vi "SAOMM-PositionGUI.vi"(0 "Hexapod VRN":refnum<visa-resource-name>="COM4", 1 "Active Refnum":refnum<vi>, 2 "PrAMS-ACK":refnum<vi>, 7 "output cluster":T1, 13 "MessageType":cluster{string[], u32[]}={["emtError", "emtAreYouThere", "emtAcknowledgment", "emtGetClientType", "emtClientType", "emtGetImageExposureTime", "emtSetImageExposureTime", "emtImageExposureTime", "emtGetOptimalExposureTime", "emtSetOptimalExposureTime", "emtOptimalExposureTime", "emtGetImageEMGain", "emtSetImageEMGain", "emtImageEMGain", "emtGetFPGACtrl", "emtSetFPGACtrl", "emtFPGACtrl", "emtGetImageWidth", "emtSetImageWidth", "emtImageWidth", "emtGetImageHeight", "emtSetImageHeight", "emtImageHeight", "emtGetImageBinning", "emtSetImageBinning", "emtImageBinning", "emtGetImageDisplayFrameRate", "emtSetImageDisplayFrameRate", "emtImageDisplayFrameRate", "emtGetROIWidth", "emtSetROIWidth", "emtROIWidth", "emtGetROIHeight", "emtSetROIHeight", "emtROIHeight", "emtGetROIXOffset", "emtSetROIXOffset", "emtROIXOffset", "emtGetROIYOffset", "emtSetROIYOffset", "emtROIYOffset", "emtStartAcquisition", "mtStopAcquisition", "emtAcquisitionStarted", "emtAcquisitionStopped", "emtGetFalconImage", "emtFalconImage"], [1, 2, 3, 4, 5, 1001, 1101, 1201, 1002, 1102, 1202, 1003, 1103, 1203, 1004, 1104, 1204, 1005, 1105, 1205, 1006, 1106, 1206, 1007, 1107, 1207, 1008, 1108, 1208, 1009, 1109, 1209, 1010, 1110, 1210, 1011, 1111, 1211, 1012, 1112, 1212, 1130, 1131, 1150, 1151, 1070, 1270]}) -> (8 "Error":bool)   [LabVIEW 2011]
uses:
  Polymorphics/Num2littleEndian(DBL).vi
panel:
  out "First Run":bool
  in  "Incrément":dbl
  in  "Incrément":dbl
  in  "V+":bool
  in  "V-":bool
  in  "U+":bool
  in  "Cancel 8":bool
  in  "Cancel 7":bool
  in  "Cancel 6":bool
  in  "Cancel 5":bool
  in  "Cancel 4":bool
  in  "Cancel 3":bool
  in  "X-":bool
  in  "keep-active":bool caption="Laisser ouvert ?"
  in  "Signature":u32=1886544237
  in  "Cancel":bool
  in  "Send":bool
  in  "X":dbl caption="Pos" format="%.4f"
  in  "Y":dbl caption="Pos" format="%.4f"
  in  "Z":dbl caption="Pos" format="%.4f"
  in  "U":dbl caption="Pos" format="%.4f"
  in  "V":dbl caption="Pos" format="%.4f"
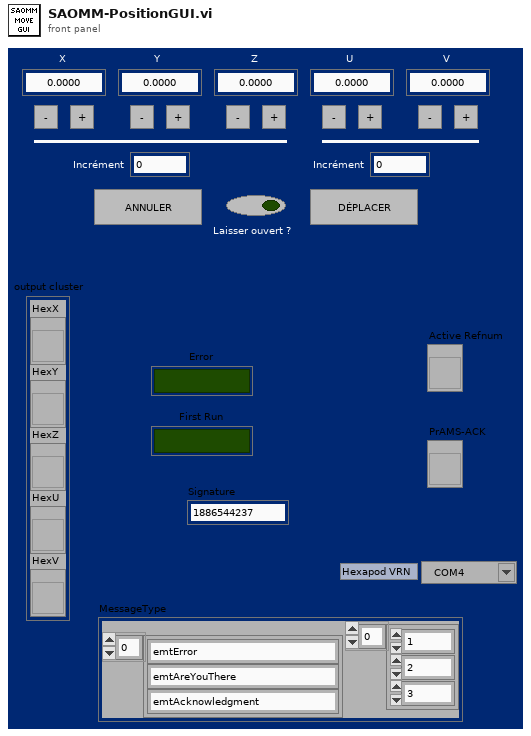
[diagram p1: front panel]
types:
  T1 = cluster{"HexX":refnum<vi>, "HexY":refnum<vi>, "HexZ":refnum<vi>, "HexU":refnum<vi>, "HexV":refnum<vi>}
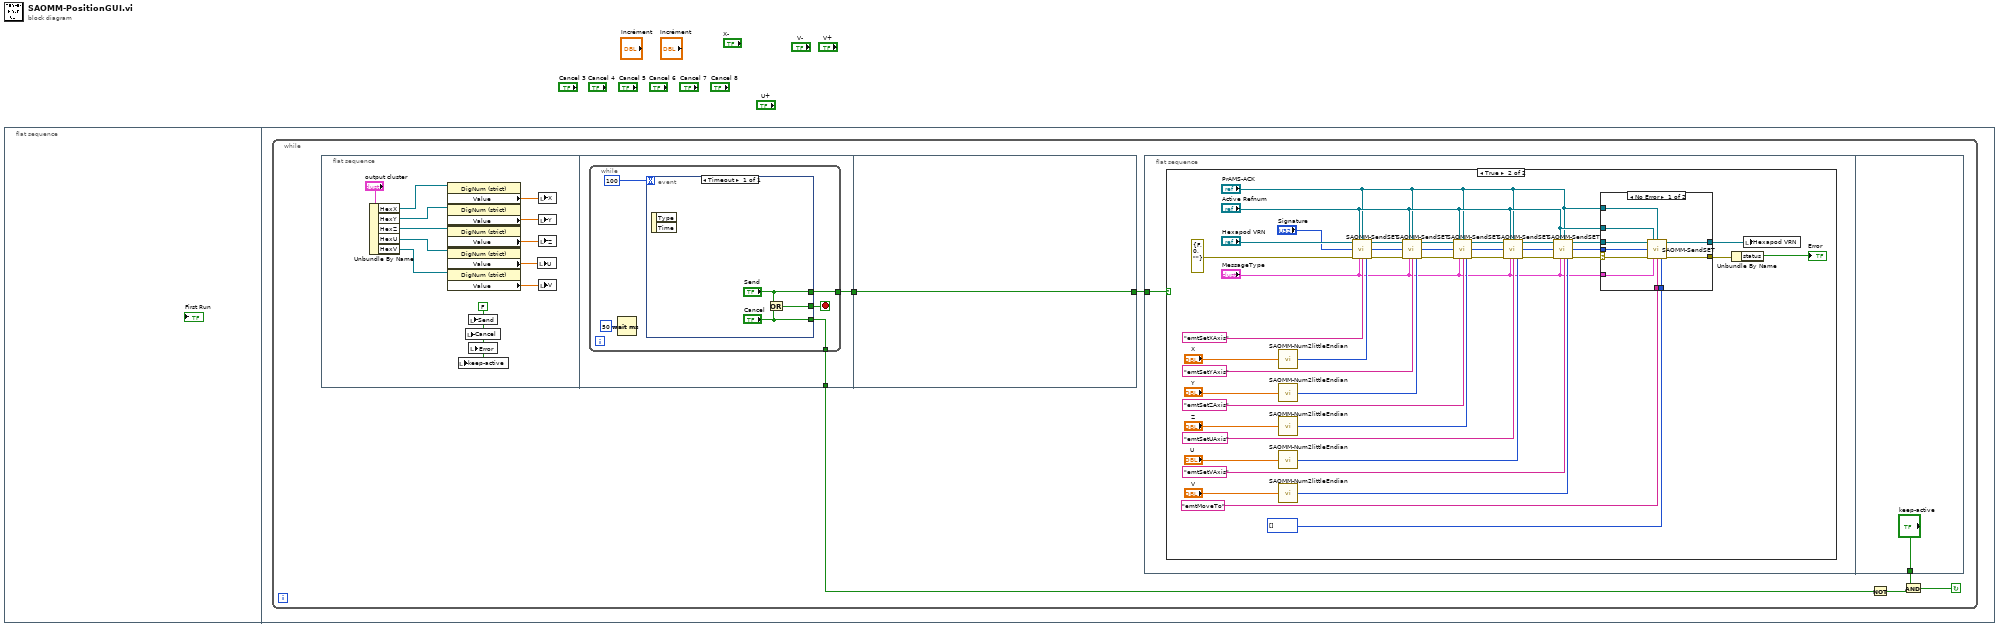
[diagram p0: block diagram]
diagram:
  n1 = flat-sequence {
    frame #0 {
    }
    frame #1 {
      n2 = while {
        stop <- w4 continue-if-true
        n3 = flat-sequence {
          tunnel: [w69] -> w2
          tunnel: [w70] -> w1
          tunnel: [w79] -> w6
          tunnel: w1 -> [w79]
          frame #0 {
            w57 = FALSE
            n4 = Unbundle By Name("output cluster") -> ("HexX"=w67:refnum<vi>, "HexY"=w66:refnum<vi>, "HexZ"=w65:refnum<vi>, "HexU"=w64:refnum<vi>, "HexV"=w63:refnum<vi>)
            n5 = property class="DigNum (strict)"(reference=w67) -> ("Value"=w58:dbl)  [unwired: 1 in, 2 out]
            n6 = property class="DigNum (strict)"(reference=w66) -> ("Value"=w59:dbl)  [unwired: 1 in, 2 out]
            n7 = property class="DigNum (strict)"(reference=w65) -> ("Value"=w60:dbl)  [unwired: 1 in, 2 out]
            n8 = property class="DigNum (strict)"(reference=w64) -> ("Value"=w61:dbl)  [unwired: 1 in, 2 out]
            n9 = property class="DigNum (strict)"(reference=w63) -> ("Value"=w62:dbl)  [unwired: 1 in, 2 out]
            n10 = local write "keep-active"(w57) -> ()
            n11 = local write "Cancel"(w57) -> ()
            n12 = local write "Send"(w57) -> ()
            n13 = local write "Error"(w57) -> ()
            n14 = local write "U"(w61) -> ()
            n15 = local write "X"(w58) -> ()
            n16 = local write "Y"(w59) -> ()
            n17 = local write "Z"(w60) -> ()
            n18 = local write "V"(w62) -> ()
          }
          frame #1 {
            n19 = while {
              tunnel: [w72] -> w70
              tunnel: [w71] -> w69
              stop <- w73 stop-if-true
              n20 = Wait (ms)(milliseconds to wait=u32 50) -> ()  [unwired: 1 out]
              n21 = event shown="[0] Timeout" {
                selector: _ -> [_]
                dyn-events: _ -> [_]
                timeout: 100 -> [_]
                tunnel: [w78] -> w73
                tunnel: ["Send"] -> w72
                tunnel: ["Cancel"] -> w71
                event Timeout {
                  n22 = event-data() -> ()  [unwired: 1 in, 2 out]
                  n23 = Or(x="Send", y="Cancel") -> (x .or. y?=w78:bool)
                }
              }
            }
          }
          frame #2 {
          }
        }
        n24 = flat-sequence {
          tunnel: w6 -> [w7]
          tunnel: ["keep-active"] -> w5
          frame #0 {
            n25 = case shown="True" w7 {
              frame False {
              }
              frame True {
                n26 = call-poly "SAOMM-Num2littleEndian.vi"("Number"="X") -> ("LiitleEndianedData"=w30:u8[])  [unwired: 14 in]
                n27 = call-poly "SAOMM-Num2littleEndian.vi"("Number"="Y") -> ("LiitleEndianedData"=w31:u8[])  [unwired: 14 in]
                n28 = call-poly "SAOMM-Num2littleEndian.vi"("Number"="Z") -> ("LiitleEndianedData"=w32:u8[])  [unwired: 14 in]
                n29 = call-poly "SAOMM-Num2littleEndian.vi"("Number"="U") -> ("LiitleEndianedData"=w35:u8[])  [unwired: 14 in]
                n30 = call-poly "SAOMM-Num2littleEndian.vi"("Number"="V") -> ("LiitleEndianedData"=w36:u8[])  [unwired: 14 in]
                n31 = call "SAOMM-SendSET.vi"("PRAMMS-COMM IN"="Hexapod VRN", "Active Refnum"="Active Refnum", "PrAMS-ACK"="PrAMS-ACK", "Signature"="Signature", "Error IN"=errorcluster {"status"=FALSE, "code"=0, "source"=""}, "MessageType"="MessageType", "Active SET"="emtSetXAxis", "Value (little endianed byte array)"=w30) -> ("PRAMMS-COMM OUT"=w21:refnum<visa-resource-name>, "Error OUT"=w27:errorcluster)  [unwired: 4 in, 2 out]
                n32 = call "SAOMM-SendSET.vi"("PRAMMS-COMM IN"=w21, "Active Refnum"="Active Refnum", "PrAMS-ACK"="PrAMS-ACK", "Signature"="Signature", "Error IN"=w27, "MessageType"="MessageType", "Active SET"="emtSetYAxis", "Value (little endianed byte array)"=w31) -> ("PRAMMS-COMM OUT"=w22:refnum<visa-resource-name>, "Error OUT"=w26:errorcluster)  [unwired: 4 in, 2 out]
                n33 = call "SAOMM-SendSET.vi"("PRAMMS-COMM IN"=w22, "Active Refnum"="Active Refnum", "PrAMS-ACK"="PrAMS-ACK", "Signature"="Signature", "Error IN"=w26, "MessageType"="MessageType", "Active SET"="emtSetZAxis", "Value (little endianed byte array)"=w32) -> ("PRAMMS-COMM OUT"=w42:refnum<visa-resource-name>, "Error OUT"=w25:errorcluster)  [unwired: 4 in, 2 out]
                n34 = call "SAOMM-SendSET.vi"("PRAMMS-COMM IN"=w42, "Active Refnum"="Active Refnum", "PrAMS-ACK"="PrAMS-ACK", "Signature"="Signature", "Error IN"=w25, "MessageType"="MessageType", "Active SET"="emtSetUAxis", "Value (little endianed byte array)"=w35) -> ("PRAMMS-COMM OUT"=w43:refnum<visa-resource-name>, "Error OUT"=w24:errorcluster)  [unwired: 4 in, 2 out]
                n35 = call "SAOMM-SendSET.vi"("PRAMMS-COMM IN"=w43, "Active Refnum"="Active Refnum", "PrAMS-ACK"="PrAMS-ACK", "Signature"="Signature", "Error IN"=w24, "MessageType"="MessageType", "Active SET"="emtSetVAxis", "Value (little endianed byte array)"=w36) -> ("PRAMMS-COMM OUT"=w41:refnum<visa-resource-name>, "Error OUT"=w40:errorcluster)  [unwired: 4 in, 2 out]
                n36 = case shown="No Error" w40 {
                  selector: w40 -> [w45 w54]
                  tunnel: "Active Refnum" -> [w53 _]
                  tunnel: "PrAMS-ACK" -> [w52 _]
                  tunnel: "Signature" -> [w51 _]
                  tunnel: [w50 w55] -> w23
                  tunnel: [w49 w54] -> w9
                  tunnel: "MessageType" -> [w48 _]
                  tunnel: "emtMoveTo" -> [w47 _]
                  tunnel: u8[] [] ("Value (little endianed byte array)") -> [w46 _]
                  tunnel: w41 -> [w44 w55]
                  frame No Error {
                    n37 = call "SAOMM-SendSET.vi"("PRAMMS-COMM IN"=w44, "Active Refnum"=w53, "PrAMS-ACK"=w52, "Signature"=w51, "Error IN"=w45, "MessageType"=w48, "Active SET"=w47, "Value (little endianed byte array)"=w46) -> ("PRAMMS-COMM OUT"=w50:refnum<visa-resource-name>, "Error OUT"=w49:errorcluster)  [unwired: 4 in, 2 out]
                  }
                  frame Error {
                  }
                }
                n38 = Unbundle By Name(w9) -> ("status"=→"Error":bool)
                n39 = local write "Hexapod VRN"(w23) -> ()
              }
            }
          }
          frame #1 {
          }
        }
        n40 = Not(x=w2) -> (.not. x?=w3:bool)
        n41 = And(x=w5, y=w3) -> (x .and. y?=w4:bool)
      }
    }
  }
